vi "Main.vi"() -> ()   [LabVIEW 2023]
uses:
  <vilib>/Instr/_visa.llb/VISA Configure Serial Port (Instr).vi
panel:
  in  "ID":u8=1
  in  "Torque Enable = 0":bool
  in  "Torque Enable = 1":bool
  in  "Send position":bool
  in  "baud rate (9600)":u32=921600
  in  "VISA resource name":refnum<visa-resource-name>
  in  "Goal Position":u32=2048
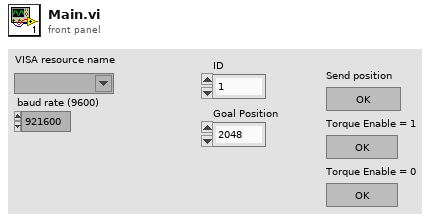
[diagram p1: front panel]
types:
  T1 = enum16{"big-endian, network order", "native, host order", "little-endian"}
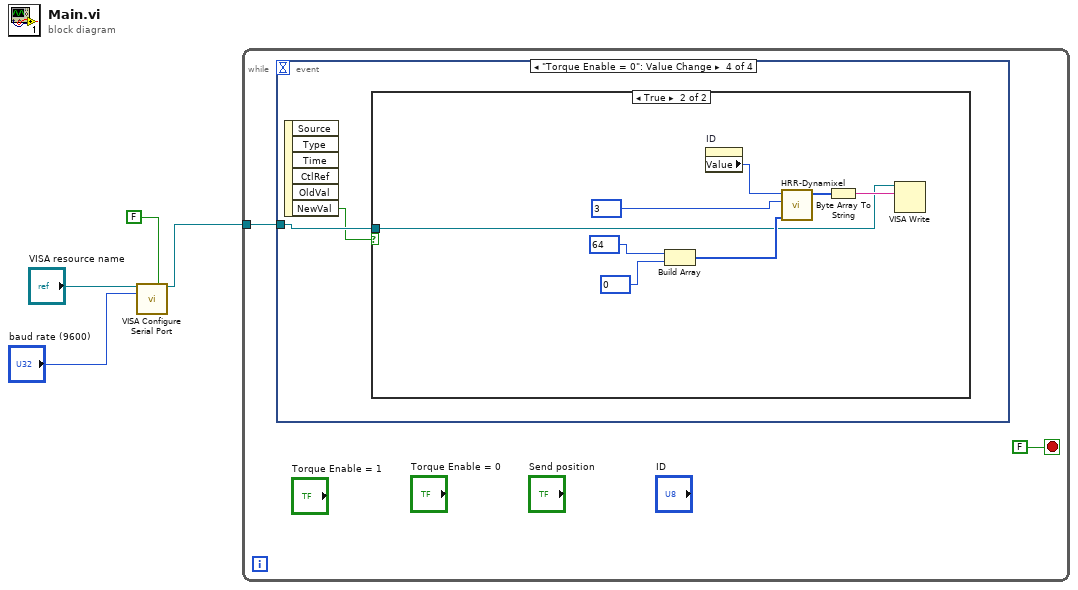
[diagram p0: block diagram]
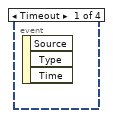
[diagram p2: hidden frame]
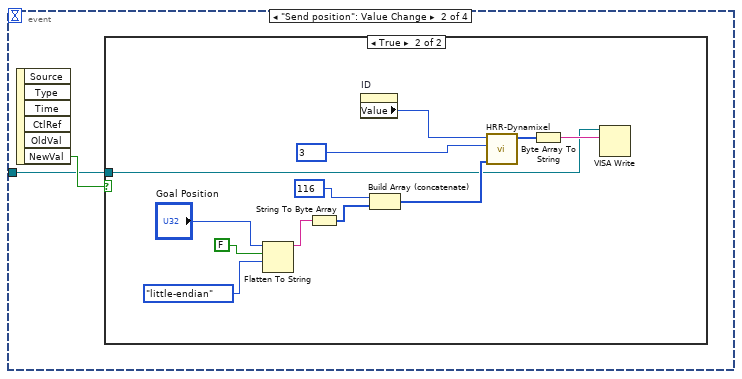
[diagram p3: hidden frame]
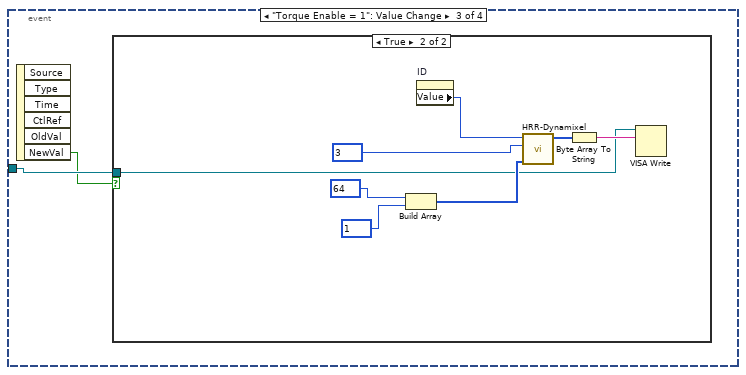
[diagram p5: hidden frame]
diagram:
  n1 = call-poly "VISA Configure Serial Port"("VISA resource name"="VISA resource name", "Enable Termination\nChar (T)"=FALSE ("Enable Termination\nChar (T)"), "baud rate (9600)"="baud rate (9600)") -> ("VISA resource name out"=w1:refnum<visa-resource-name>)  [unwired: 11 in, 1 out]
  n2 = while {
    tunnel: w1 -> [w6]
    stop <- FALSE stop-if-true
    n3 = event shown="[3] \"Torque Enable = 0\": Value Change" {
      selector: _ -> [_ _ _ _]
      dyn-events: _ -> [_ _ _ _]
      timeout: _ -> [_ _ _ _]
      tunnel: w6 -> [_ w7 w22 w32]
      event Timeout {
        n4 = event-data() -> ()  [unwired: 1 in, 3 out]
      }
      event "Send position": Value Change {
        n5 = event-data() -> ("NewVal"=w8:bool)  [unwired: 1 in, 5 out]
        n6 = case shown="True" w8 {
          tunnel: w7 -> [_ w10]
          frame False {
          }
          frame True {
            n7 = Flatten To String(anything="Goal Position", prepend array or string size? (T)=FALSE, byte order (0:big-endian, network order)=T1."little-endian") -> (data string=w15:string)  [unwired: 1 in, 2 out]
            n8 = String To Byte Array(string=w15) -> (unsigned byte array=w16:u8[])
            n9 = property on="ID" class="DigNum (strict)"() -> ("Value"=w9:u8)  [unwired: 2 in, 2 out]
            n10 = Build Array (concatenate)(u8 116 ("Instruction"), w16) -> (w17:u8[])
            n11 = call "HRR-Dynamixel.vi"("ID"=w9, "Instruction"=u8 3, "Array in"=w17) -> ("Array out"=w19:u8[])  [unwired: 7 in]
            n12 = Byte Array To String(unsigned byte array=w19) -> (string=w20:string)
            n13 = VISA Write(VISA resource name=w10, write buffer=w20) -> ()  [unwired: 1 in, 3 out]
          }
        }
      }
      event "Torque Enable = 1": Value Change {
        n14 = event-data() -> ("NewVal"=w21:bool)  [unwired: 1 in, 5 out]
        n15 = case shown="True" w21 {
          tunnel: w22 -> [_ w25]
          frame False {
          }
          frame True {
            n16 = Build Array(u8 64 ("Instruction"), u8 1 ("Instruction")) -> (w30:u8[])
            n17 = property on="ID" class="DigNum (strict)"() -> ("Value"=w23:u8)  [unwired: 2 in, 2 out]
            n18 = call "HRR-Dynamixel.vi"("ID"=w23, "Instruction"=u8 3, "Array in"=w30) -> ("Array out"=w29:u8[])  [unwired: 7 in]
            n19 = Byte Array To String(unsigned byte array=w29) -> (string=w28:string)
            n20 = VISA Write(VISA resource name=w25, write buffer=w28) -> ()  [unwired: 1 in, 3 out]
          }
        }
      }
      event "Torque Enable = 0": Value Change {
        n21 = event-data() -> ("NewVal"=w31:bool)  [unwired: 1 in, 5 out]
        n22 = case shown="True" w31 {
          tunnel: w32 -> [_ w35]
          frame False {
          }
          frame True {
            n23 = Build Array(u8 64 ("Instruction"), u8 0 ("Instruction")) -> (w40:u8[])
            n24 = property on="ID" class="DigNum (strict)"() -> ("Value"=w33:u8)  [unwired: 2 in, 2 out]
            n25 = call "HRR-Dynamixel.vi"("ID"=w33, "Instruction"=u8 3, "Array in"=w40) -> ("Array out"=w39:u8[])  [unwired: 7 in]
            n26 = Byte Array To String(unsigned byte array=w39) -> (string=w38:string)
            n27 = VISA Write(VISA resource name=w35, write buffer=w38) -> ()  [unwired: 1 in, 3 out]
          }
        }
      }
    }
  }
